vi "Test Flatten.vi"() -> ()   [LabVIEW 2021]
uses:
  CIF_NIChn_FifoCAN.lvclass
  ChannelCommon/typedef/Datatype CAN.ctl
  ChannelCommon/ChannelCommon.lvlib
  ChannelCommon/typedef/FIFO Header.ctl
  ChannelCommon/typedef/TimeStamps.ctl
panel:
  in  "FIFO Timestamps":T1
  out "Data":T2[](array[typedef]) {"Tags" format="%.0x"; "payload" format="%x"; "identifier" format="%x"}
  in  "CAN Data":T2[](array[typedef])=[{"payload"=[0, 0, 0, 0, 0, 0, 2, 51], "identifier"=291, "Tags"=0, "Timestamp"=0}, {"payload"=[0, 0, 0, 0, 0, 0, 2, 51], "identifier"=291, "Tags"=0, "Timestamp"=0}] {"Tags" format="%.0x"; "payload" format="%x"; "identifier" format="%x"}
  out "Header":T3={"Length"=52, "T0"=321, "T_Out"=123, "T_Tx"=1724093393726059437, "Ctr"=1, "ClockID"=0}
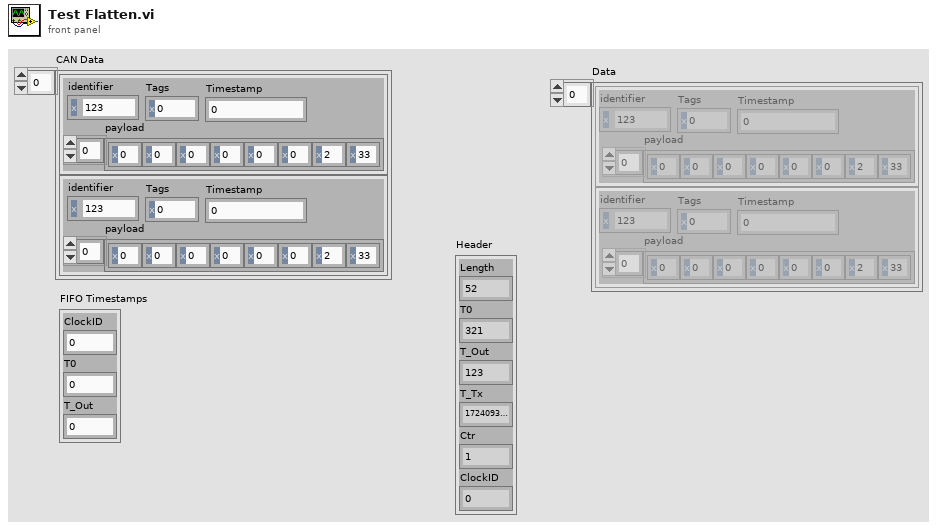
[diagram p1: front panel]
types:
  T1 = typedef "ChannelCommon.lvlib/TimeStamps.ctl" = cluster{"ClockID":u8, "T0":u64, "T_Out":u64}
  T2 = typedef "ChannelCommon.lvlib/Datatype CAN.ctl" = cluster{"payload":u8[], "identifier":u32, "Tags":u8, "Timestamp":u64}
  T3 = typedef "ChannelCommon.lvlib/FIFO Header.ctl" = cluster{"Length":u64, "T0":i64, "T_Out":i64, "T_Tx":i64, "Ctr":u64, "ClockID":u8}
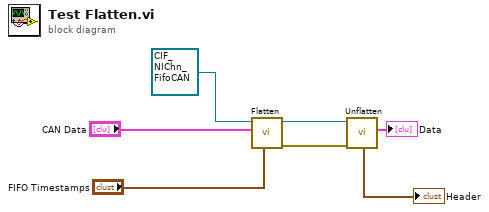
[diagram p0: block diagram]
diagram:
  n1 = call "Flatten.vi"("FIFO Timestamps"="FIFO Timestamps", "Data in"="CAN Data", "CIFTag in"=refnum<class "CIF_NIChn_FifoCAN.lvclass"> refnum) -> ("error out"=w6:errorcluster, "CIFTag out"=w7:refnum<class "CIF_NIChn_FifoCAN.lvclass">)  [unwired: 6 in, 1 out]
  n2 = call "Unflatten.vi"("error in (no error)"=w6, "CIFFifoCAN in"=w7) -> ("Data"=→"Data":T2[], "Header"=→"Header":T3)  [unwired: 6 in, 2 out]
